vi "getRfRampData.vi"(8 "error in (no error)":errorcluster, 11 "RfRamp in":refnum<class "RfRamp.lvclass">) -> (0 "error out":errorcluster, 2 "Array":T1(array[cluster]), 3 "RfRamp out":refnum<class "RfRamp.lvclass">)   [LabVIEW 2009, in "Tools.lvlib" / "Scripting.lvlib" / "RfRamp.lvclass"]
uses:
  RfRamp.lvclass
  DatabaseHelpers/Database Objects/Channel/RfOutputChannel/RfOutputChannel.lvclass
  RfRamp.lvclass/RfRamp.ctl
  ScriptEvent.lvclass
  xmlNode/xmlNode.lvclass
  Rf Event/rf.lvclass
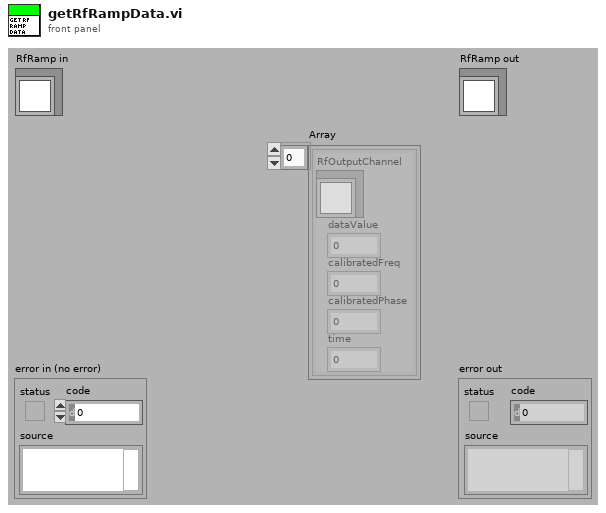
[diagram p1: front panel]
types:
  T1 = cluster{"RfOutputChannel":refnum<class "RfOutputChannel.lvclass">, "dataValue":dbl, "calibratedFreq":dbl, "calibratedPhase":dbl, "time":dbl}[]
  T2 = cluster{"RfOutputChannel":refnum<class "RfOutputChannel.lvclass">, "dataValue":dbl, "calibratedFreq":dbl, "calibratedPhase":dbl, "time":dbl}
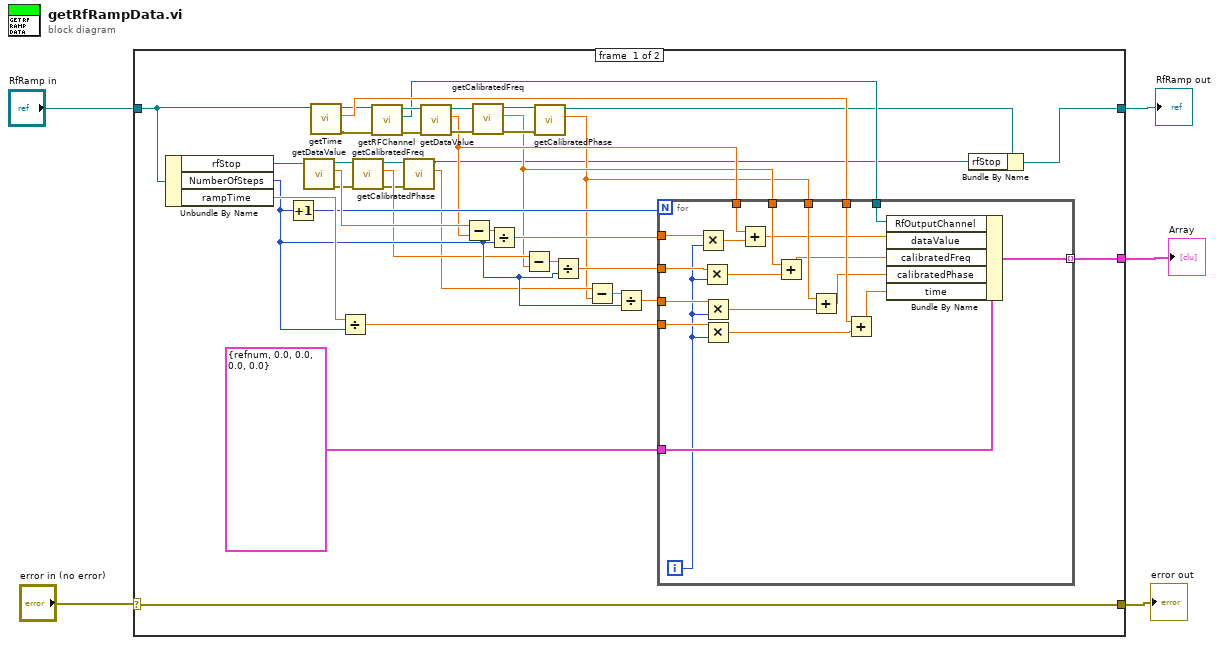
[diagram p0: block diagram]
diagram:
  n1 = case shown="No Error" "error in (no error)" {
    selector: "error in (no error)" -> [w40 w65]
    tunnel: [w40 w65] -> w4
    tunnel: [w8 w64] -> w1
    tunnel: "RfRamp in" -> [w43 w64]
    tunnel: [w9 _] -> w2
    frame #0 {
      n2 = Unbundle By Name(w43) -> ("rfStop"=w42:refnum<class "rf.lvclass">, "NumberOfSteps"=w31:i32, "rampTime"=w41:dbl)
      n3 = Increment(x=w31) -> (x+1=w32:i32)
      n4 = call "getDataValue.vi"("ScriptEvent.lvclass in"=w42) -> ("error out"=w25:errorcluster, "dataValue"=w39:dbl, "ScriptEvent.lvclass out"=w26:refnum<class "rf.lvclass">)  [unwired: 8 in]
      n5 = call "getTime.vi"("ScriptEvent.lvclass in"=w43) -> ("error out"=w11:errorcluster, "time"=w16:dbl, "ScriptEvent.lvclass out"=w15:refnum<class "RfRamp.lvclass">)  [unwired: 8 in]
      n6 = Divide(x=w41, y=w31) -> (x/y=w30:dbl)
      n7 = call "getCalibratedFreq.vi"("error in (no error)"=w25, "rf in"=w26) -> ("error out"=w22:errorcluster, "calibratedFreq"=w24:dbl, "rf out"=w23:refnum<class "rf.lvclass">)  [unwired: 7 in]
      n8 = call "getRFChannel.vi"("error in (no error)"=w11, "rf.lvclass in"=w15) -> ("error out"=w12:errorcluster, "RfOutputChannel.lvclass"=w10:refnum<class "RfOutputChannel.lvclass">, "rf.lvclass out"=w14:refnum<class "RfRamp.lvclass">)  [unwired: 7 in]
      n9 = call "getCalibratedPhase.vi"("error in (no error)"=w22, "rf in"=w23) -> ("calibratedPhase"=w21:dbl, "rf out"=w6:refnum<class "rf.lvclass">)  [unwired: 7 in, 1 out]
      n10 = call "getDataValue.vi"("error in (no error)"=w12, "ScriptEvent.lvclass in"=w14) -> ("error out"=w29:errorcluster, "dataValue"=w19:dbl, "ScriptEvent.lvclass out"=w13:refnum<class "RfRamp.lvclass">)  [unwired: 7 in]
      n11 = Subtract(x=w39, y=w19) -> (x-y=w38:dbl)
      n12 = call "getCalibratedFreq.vi"("error in (no error)"=w29, "rf in"=w13) -> ("error out"=w27:errorcluster, "calibratedFreq"=w18:dbl, "rf out"=w28:refnum<class "RfRamp.lvclass">)  [unwired: 7 in]
      n13 = Divide(x=w38, y=w31) -> (x/y=w37:dbl)
      n14 = Subtract(x=w24, y=w18) -> (x-y=w36:dbl)
      n15 = call "getCalibratedPhase.vi"("error in (no error)"=w27, "rf in"=w28) -> ("calibratedPhase"=w17:dbl, "rf out"=w7:refnum<class "RfRamp.lvclass">)  [unwired: 7 in, 1 out]
      n16 = Divide(x=w36, y=w31) -> (x/y=w35:dbl)
      n17 = Subtract(x=w21, y=w17) -> (x-y=w34:dbl)
      n18 = Divide(x=w34, y=w31) -> (x/y=w33:dbl)
      n19 = for {
        N: w32 -> [_]
        tunnel: w37 -> [w62]
        tunnel: w35 -> [w61]
        tunnel: w33 -> [w60]
        tunnel: w30 -> [w59]
        tunnel: T2 {"RfOutputChannel"=refnum, "dataValue"=0.0, "calibratedFreq"=0.0, "calibratedPhase"=0.0, "time"=0.0} ("data") -> [w63]
        tunnel: w19 -> [w56]
        tunnel: w18 -> [w55]
        tunnel: w17 -> [w52]
        tunnel: w16 -> [w50]
        tunnel: w10 -> [w45]
        tunnel: [w44] -> w9 mode=indexing
        i -> [w58]
        n20 = Multiply(x=w62, y=w58) -> (x*y=w57:dbl)
        n21 = Multiply(x=w61, y=w58) -> (x*y=w54:dbl)
        n22 = Multiply(x=w60, y=w58) -> (x*y=w53:dbl)
        n23 = Multiply(x=w59, y=w58) -> (x*y=w51:dbl)
        n24 = Add(x=w56, y=w57) -> (x+y=w49:dbl)
        n25 = Add(x=w55, y=w54) -> (x+y=w48:dbl)
        n26 = Add(x=w52, y=w53) -> (x+y=w47:dbl)
        n27 = Add(x=w50, y=w51) -> (x+y=w46:dbl)
        n28 = Bundle By Name(cluster=w63, "RfOutputChannel"=w45, "dataValue"=w49, "calibratedFreq"=w48, "calibratedPhase"=w47, "time"=w46) -> (w44:T2)
      }
      n29 = Bundle By Name(cluster=w7, "rfStop"=w6) -> (w8:refnum<class "RfRamp.lvclass">)
    }
    frame #1 {
    }
  }
  "error out" <- w4
  "RfRamp out" <- w1
  "Array" <- w2
